vi "2D plot_take linecut.vi"() -> ()   [LabVIEW 2016]
uses:
  <vilib>/Analysis/baseanly.llb/Mean (DBL).vi
  <vilib>/Analysis/NI_AALPro.lvlib
  <vilib>/Analysis/NI_AALBase.lvlib
panel:
  in  "Tab Control":enum32{"Page 1", "Page 2"}(tab)=enum."Page 2"
  in  "E 5":dbl[][](graph)
  in  "Array":i32[](array[numeric])=[0, 1]
  in  "cond":dbl[][](graph)
  out "E 4":dbl[][](graph)
  out "Data 4":cluster{dbl[], dbl[]}(graph)
  out "Data 5":cluster{dbl[], dbl[]}[](graph)
  out "Intensity Graph 15":dbl[][](graph)
  in  "alpha":dbl format="%#_13g"
  # "29.2    .139\n60.4    .129"
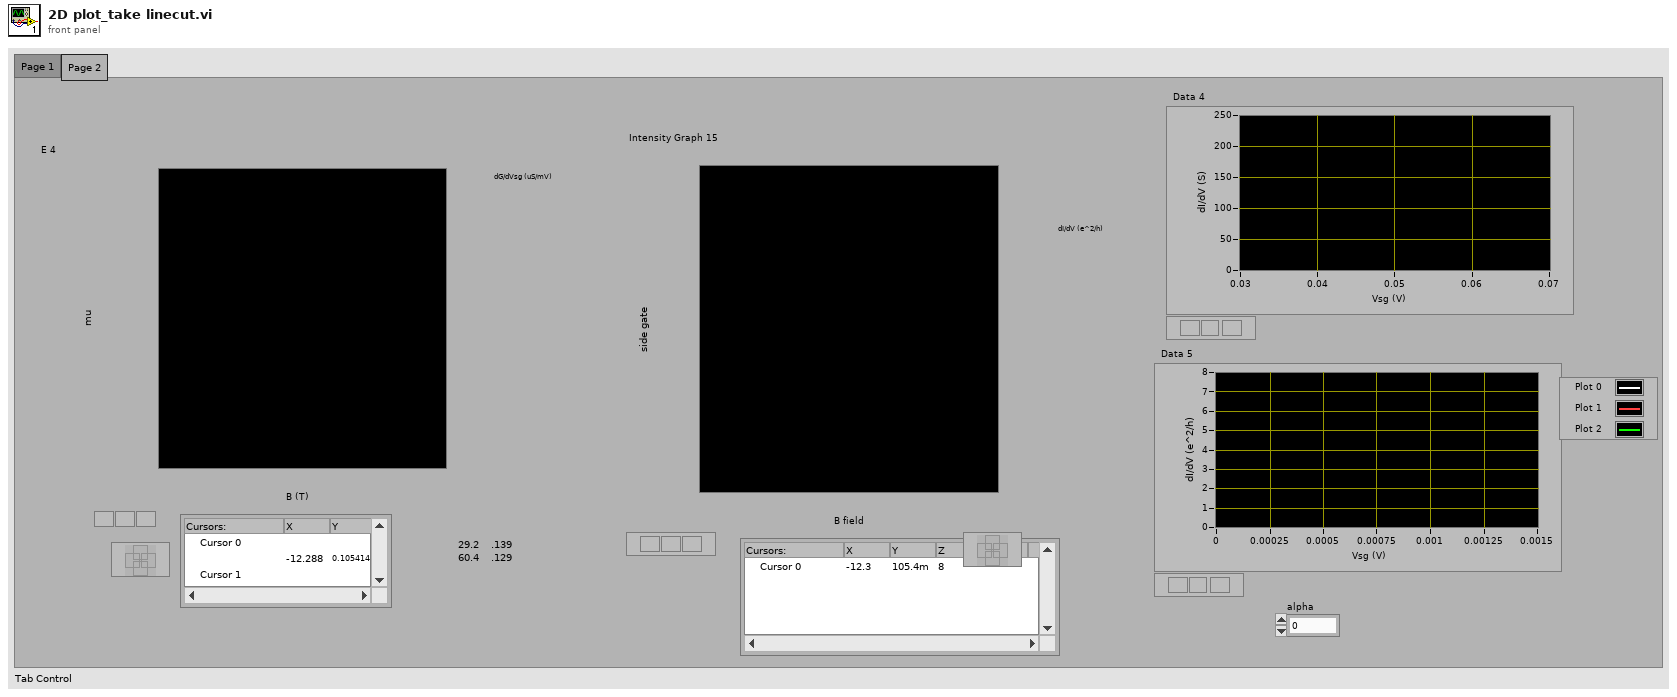
[diagram p1: front panel]
types:
  T1 = typedef "LVPointDoubleTypeDef.ctl" = cluster{"Cursor X":dbl, "Cursor Y":dbl}
  T2 = typedef "LVOffsetAndMultiplierTypeDef.ctl" = cluster{"Offset":dbl, "Multiplier":dbl}
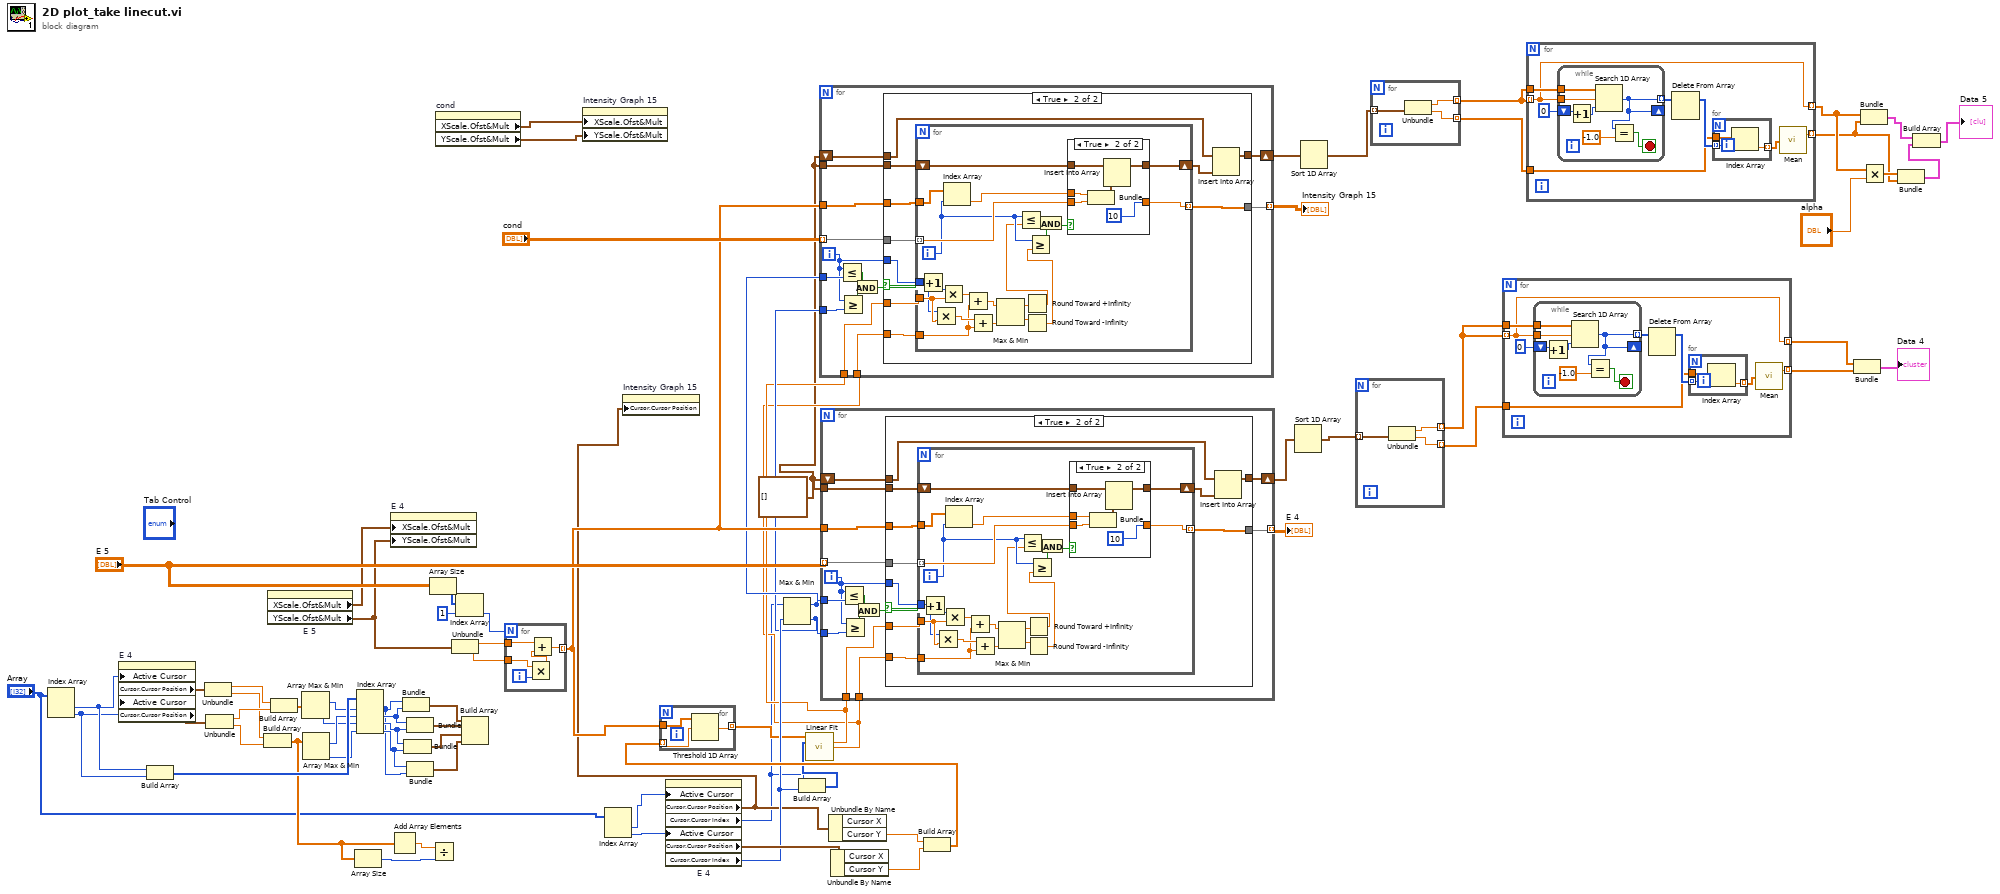
[diagram p0: block diagram]
diagram:
  w17 = cluster{dbl, dbl}[] []
  n1 = Index Array(array="Array") -> (element #1=w51:i32, element #2=w50:i32)  [unwired: 2 in]
  n2 = property on="E 4" class="IntGraph (strict)"("Active Cursor"=w51, "Active Cursor"=w50) -> ("Cursor.Cursor Position"=w74:T1, "Cursor.Cursor Position"=w73:T1)  [unwired: 2 in, 2 out]
  n3 = Build Array(w51, w50) -> (w69:i32[])
  n4 = Unbundle(w74) -> ("Cursor X"=w72:dbl, "Cursor Y"=w67:dbl)
  n5 = Unbundle(w73) -> ("Cursor X"=w71:dbl, "Cursor Y"=w68:dbl)
  n6 = Build Array(w67, w68) -> (w53:dbl[])
  n7 = property on="E 5" class="IntGraph (strict)"() -> ("XScale.Ofst&Mult"=w25:T2, "YScale.Ofst&Mult"=w24:T2)  [unwired: 2 in, 2 out]
  n8 = Build Array(w72, w71) -> (w70:dbl[])
  n9 = Array Max & Min(array=w70) -> (max index (indices)=w66:i32, min index (indices)=w64:i32)  [unwired: 2 out]
  n10 = Array Max & Min(array=w53) -> (max index (indices)=w65:i32, min index (indices)=w63:i32)  [unwired: 2 out]
  n11 = Array Size(array=w53) -> (size(s)=w52:i32)
  n12 = Index Array(array=w69, index #1=w66, index #2=w65, index #3=w64, index #4=w63) -> (element #1=w59:i32, element #2=w62:i32, element #3=w61:i32, element #4=w60:i32)
  n13 = property on="E 4" class="IntGraph (strict)"("XScale.Ofst&Mult"=w25, "YScale.Ofst&Mult"=w24) -> ()  [unwired: 2 in, 2 out]
  n14 = Add Array Elements(numeric array=w53) -> (sum=w54:dbl)
  n15 = Bundle(w59, w62) -> (w58:cluster{i32, i32})  [unwired: 1 in]
  n16 = Bundle(w61, w60) -> (w56:cluster{i32, i32})  [unwired: 1 in]
  n17 = Bundle(w62, w61) -> (w57:cluster{i32, i32})  [unwired: 1 in]
  n18 = Bundle(w60, w59) -> (w55:cluster{i32, i32})  [unwired: 1 in]
  n19 = Array Size(array="E 5") -> (size(s)=w47:i32[])
  n20 = Divide(x=w54, y=w52) -> ()  [unwired: 1 out]
  n21 = property on="cond" class="IntGraph (strict)"() -> ("XScale.Ofst&Mult"=w2:T2, "YScale.Ofst&Mult"=w1:T2)  [unwired: 2 in, 2 out]
  n22 = Unbundle(w24) -> ("Offset"=w49:dbl, "Multiplier"=w48:dbl)
  n23 = Index Array(array=w47, index=1) -> (element=w44:i32)
  n24 = Build Array(w58, w57, w56, w55) -> ()  [unwired: 1 out]
  n25 = for {
    N: w44 -> [_]
    tunnel: w49 -> [w78]
    tunnel: w48 -> [w77]
    tunnel: [w75] -> w22 mode=indexing
    i -> [w79]
    n26 = Multiply(x=w77, y=w79) -> (x*y=w76:dbl)
    n27 = Add(x=w78, y=w76) -> (x+y=w75:dbl)
  }
  n28 = property on="Intensity Graph 15" class="IntGraph (strict)"("XScale.Ofst&Mult"=w2, "YScale.Ofst&Mult"=w1) -> ()  [unwired: 2 in, 2 out]
  n29 = Index Array(array="Array") -> (element #1=w34:i32, element #2=w33:i32)  [unwired: 2 in]
  n30 = property on="E 4" class="IntGraph (strict)"("Active Cursor"=w34, "Active Cursor"=w33) -> ("Cursor.Cursor Position"=w11:T1, "Cursor.Cursor Index"=w10:i32, "Cursor.Cursor Position"=w41:T1, "Cursor.Cursor Index"=w37:i32)  [unwired: 2 in, 2 out]
  n31 = property on="Intensity Graph 15" class="IntGraph (strict)"("Cursor.Cursor Position"=w11) -> ()  [unwired: 2 in, 2 out]
  n32 = Max & Min(x=w10, y=w37) -> (max(x,y)=w21:i32, min(x,y)=w20:i32)
  n33 = Build Array(w10, w37) -> (w36:i32[])
  n34 = Unbundle By Name(w11) -> ("Cursor Y"=w40:dbl)  [unwired: 1 out]
  n35 = Unbundle By Name(w41) -> ("Cursor Y"=w39:dbl)  [unwired: 1 out]
  n36 = Build Array(w40, w39) -> (w38:dbl[])
  n37 = for {
    tunnel: w22 -> [w82]
    tunnel: w38 -> [w81] mode=indexing
    tunnel: [w80] -> w35 mode=indexing
    n38 = Threshold 1D Array(2:w81, 3:w82) -> (0:w80:dbl)  [unwired: 1 in]
  }
  n39 = call <vilib>:"Linear Fit.vi"("Y"=w35, "X"=w36) -> ("slope"=w19:dbl, "intercept"=w18:dbl)  [unwired: 9 in, 3 out]
  n40 = for {
    tunnel: w21 -> [w93]
    tunnel: w20 -> [w92]
    tunnel: w19 -> [w89]
    tunnel: w18 -> [w88]
    tunnel: "cond" -> [w91] mode=indexing
    tunnel: [w90] -> w16 mode=indexing
    tunnel: w22 -> [w86]
    shift-right: [w85] -> w15
    shift-left: w17 -> [w84]
    tunnel: w17 -> [w83]
    i -> [w87]
    n41 = Less Or Equal?(x=w87, y=w93) -> (x <= y?=w95:bool)
    n42 = Greater Or Equal?(x=w87, y=w92) -> (x >= y?=w94:bool)
    n43 = And(x=w95, y=w94) -> (x .and. y?=w96:bool)
    n44 = case shown="True" w96 {
      tunnel: w91 -> [w98 w105]
      tunnel: [w98 w104] -> w90
      tunnel: w89 -> [_ w108]
      tunnel: w87 -> [_ w107]
      tunnel: w88 -> [_ w106]
      tunnel: w86 -> [_ w103]
      tunnel: [w97 w102] -> w85
      tunnel: w84 -> [w97 w101]
      tunnel: w83 -> [_ w100]
      frame False {
      }
      frame True {
        n45 = for {
          tunnel: w108 -> [w127]
          tunnel: w107 -> [w124]
          tunnel: w106 -> [w126]
          tunnel: w105 -> [w130] mode=indexing
          tunnel: [w129] -> w104 mode=indexing
          tunnel: w103 -> [w122]
          shift-right: [w116] -> w99
          shift-left: w100 -> [w115]
          i -> [w121]
          n46 = Increment(x=w124) -> (x+1=w123:i32)
          n47 = Multiply(x=w124, y=w127) -> (x*y=w128:dbl)
          n48 = Multiply(x=w123, y=w127) -> (x*y=w125:dbl)
          n49 = Index Array(array=w122, index=w121) -> (element=w120:dbl)
          n50 = Add(x=w125, y=w126) -> (x+y=w114:dbl)
          n51 = Add(x=w128, y=w126) -> (x+y=w113:dbl)
          n52 = Max & Min(x=w114, y=w113) -> (max(x,y)=w112:dbl, min(x,y)=w111:dbl)
          n53 = Round Toward +Infinity(x=w112) -> (ceil(x): smallest int >= x=w110:dbl)
          n54 = Less Or Equal?(x=w121, y=w110) -> (x <= y?=w119:bool)
          n55 = Round Toward -Infinity(1:w111) -> (0:w109:dbl)
          n56 = Greater Or Equal?(x=w121, y=w109) -> (x >= y?=w118:bool)
          n57 = And(x=w119, y=w118) -> (x .and. y?=w117:bool)
          n58 = case shown="True" w117 {
            tunnel: w130 -> [w132 w136]
            tunnel: [w132 10] -> w129
            tunnel: w120 -> [_ w137]
            tunnel: [w131 w134] -> w116
            tunnel: w115 -> [w131 w133]
            frame False {
            }
            frame True {
              n59 = Bundle(w137, w136) -> (w135:cluster{dbl, dbl})  [unwired: 1 in]
              n60 = Insert Into Array(array=w133, new element=w135) -> (w134:cluster{dbl, dbl}[])  [unwired: 1 in]
            }
          }
        }
        n61 = Insert Into Array(array=w101, new element=w99) -> (w102:cluster{dbl, dbl}[])  [unwired: 1 in]
      }
    }
  }
  "Intensity Graph 15" <- w16
  n62 = for {
    tunnel: w21 -> [w149]
    tunnel: w20 -> [w148]
    tunnel: w19 -> [w145]
    tunnel: w18 -> [w144]
    tunnel: "E 5" -> [w147] mode=indexing
    tunnel: [w146] -> w43 mode=indexing
    tunnel: w22 -> [w142]
    shift-right: [w141] -> w32
    shift-left: w17 -> [w140]
    tunnel: w17 -> [w139]
    i -> [w143]
    n63 = Less Or Equal?(x=w143, y=w149) -> (x <= y?=w151:bool)
    n64 = Greater Or Equal?(x=w143, y=w148) -> (x >= y?=w150:bool)
    n65 = And(x=w151, y=w150) -> (x .and. y?=w152:bool)
    n66 = case shown="True" w152 {
      tunnel: w147 -> [w154 w161]
      tunnel: [w154 w160] -> w146
      tunnel: w145 -> [_ w164]
      tunnel: w143 -> [_ w163]
      tunnel: w144 -> [_ w162]
      tunnel: w142 -> [_ w159]
      tunnel: [w153 w158] -> w141
      tunnel: w140 -> [w153 w157]
      tunnel: w139 -> [_ w156]
      frame False {
      }
      frame True {
        n67 = for {
          tunnel: w164 -> [w183]
          tunnel: w163 -> [w180]
          tunnel: w162 -> [w182]
          tunnel: w161 -> [w186] mode=indexing
          tunnel: [w185] -> w160 mode=indexing
          tunnel: w159 -> [w178]
          shift-right: [w172] -> w155
          shift-left: w156 -> [w171]
          i -> [w177]
          n68 = Increment(x=w180) -> (x+1=w179:i32)
          n69 = Multiply(x=w180, y=w183) -> (x*y=w184:dbl)
          n70 = Multiply(x=w179, y=w183) -> (x*y=w181:dbl)
          n71 = Index Array(array=w178, index=w177) -> (element=w176:dbl)
          n72 = Add(x=w181, y=w182) -> (x+y=w170:dbl)
          n73 = Add(x=w184, y=w182) -> (x+y=w169:dbl)
          n74 = Max & Min(x=w170, y=w169) -> (max(x,y)=w168:dbl, min(x,y)=w167:dbl)
          n75 = Round Toward +Infinity(x=w168) -> (ceil(x): smallest int >= x=w166:dbl)
          n76 = Less Or Equal?(x=w177, y=w166) -> (x <= y?=w175:bool)
          n77 = Round Toward -Infinity(1:w167) -> (0:w165:dbl)
          n78 = Greater Or Equal?(x=w177, y=w165) -> (x >= y?=w174:bool)
          n79 = And(x=w175, y=w174) -> (x .and. y?=w173:bool)
          n80 = case shown="True" w173 {
            tunnel: w186 -> [w188 w192]
            tunnel: [w188 10] -> w185
            tunnel: w176 -> [_ w193]
            tunnel: [w187 w190] -> w172
            tunnel: w171 -> [w187 w189]
            frame False {
            }
            frame True {
              n81 = Bundle(w193, w192) -> (w191:cluster{dbl, dbl})  [unwired: 1 in]
              n82 = Insert Into Array(array=w189, new element=w191) -> (w190:cluster{dbl, dbl}[])  [unwired: 1 in]
            }
          }
        }
        n83 = Insert Into Array(array=w157, new element=w155) -> (w158:cluster{dbl, dbl}[])  [unwired: 1 in]
      }
    }
  }
  "E 4" <- w43
  n84 = Sort 1D Array(array=w32) -> (sorted array=w31:cluster{dbl, dbl}[])
  n85 = Sort 1D Array(array=w15) -> (sorted array=w14:cluster{dbl, dbl}[])
  n86 = for {
    tunnel: w31 -> [w197] mode=indexing
    tunnel: [w196] -> w30 mode=indexing
    tunnel: [w195] -> w29 mode=indexing
    n87 = Unbundle(w197) -> (w196:dbl, w195:dbl)
  }
  n88 = for {
    tunnel: w14 -> [w200] mode=indexing
    tunnel: [w199] -> w13 mode=indexing
    tunnel: [w198] -> w12 mode=indexing
    n89 = Unbundle(w200) -> (w199:dbl, w198:dbl)
  }
  n90 = for {
    tunnel: w30 -> [w206]
    tunnel: w30 -> [w201] mode=indexing
    tunnel: w29 -> [w203]
    tunnel: [w202] -> w28 mode=indexing
    tunnel: [w201] -> w27 mode=indexing
    n91 = while {
      tunnel: w206 -> [w218]
      tunnel: w201 -> [w217]
      shift-right: [w212] -> _
      shift-left: 0 ("index of element") -> [w214]
      tunnel: [w212] -> w207 mode=indexing
      stop <- w215 stop-if-true
      n92 = Increment(x=w214) -> (x+1=w213:i32)
      n93 = Search 1D Array(1D array=w218, element=w217, start index (0)=w213) -> (index of element=w212:i32)
      n94 = Equal?(x=w212, y=-1.0) -> (x = y?=w215:bool)
    }
    n95 = Delete From Array(array=w207) -> (array with subset deleted=w205:i32[])  [unwired: 2 in, 1 out]
    n96 = for {
      tunnel: w203 -> [w211]
      tunnel: w205 -> [w210] mode=indexing
      tunnel: [w209] -> w204 mode=indexing
      n97 = Index Array(array=w211, index=w210) -> (element=w209:dbl)
    }
    n98 = call-poly <vilib>:"Mean.vi"("X"=w204) -> ("mean"=w202:dbl)  [unwired: 1 out]
  }
  n99 = for {
    tunnel: w13 -> [w224]
    tunnel: w13 -> [w219] mode=indexing
    tunnel: w12 -> [w221]
    tunnel: [w220] -> w4 mode=indexing
    tunnel: [w219] -> w7 mode=indexing
    n100 = while {
      tunnel: w224 -> [w236]
      tunnel: w219 -> [w235]
      shift-right: [w230] -> _
      shift-left: 0 ("index of element") -> [w232]
      tunnel: [w230] -> w225 mode=indexing
      stop <- w233 stop-if-true
      n101 = Increment(x=w232) -> (x+1=w231:i32)
      n102 = Search 1D Array(1D array=w236, element=w235, start index (0)=w231) -> (index of element=w230:i32)
      n103 = Equal?(x=w230, y=-1.0) -> (x = y?=w233:bool)
    }
    n104 = Delete From Array(array=w225) -> (array with subset deleted=w223:i32[])  [unwired: 2 in, 1 out]
    n105 = for {
      tunnel: w221 -> [w229]
      tunnel: w223 -> [w228] mode=indexing
      tunnel: [w227] -> w222 mode=indexing
      n106 = Index Array(array=w229, index=w228) -> (element=w227:dbl)
    }
    n107 = call-poly <vilib>:"Mean.vi"("X"=w222) -> ("mean"=w220:dbl)  [unwired: 1 out]
  }
  n108 = Bundle(w27, w28) -> (→"Data 4":cluster{dbl[], dbl[]})  [unwired: 1 in]
  n109 = Bundle(w7, w4) -> (w9:cluster{dbl[], dbl[]})  [unwired: 1 in]
  n110 = Multiply(x=w7, y="alpha") -> (x*y=w5:dbl[])
  n111 = Bundle(w5, w4) -> (w3:cluster{dbl[], dbl[]})  [unwired: 1 in]
  n112 = Build Array(w9, w3) -> (→"Data 5":cluster{dbl[], dbl[]}[])
